vi "Host.vi"() -> ()   [LabVIEW 2018]
uses:
  <vilib>/userdefined/High Color/nirio_resource_hc.ctl
  <instrlib>/niDCPower/nidcpower.llb/niDCPower Measurement Type.ctl
  <vilib>/FPGAPlugInAG/PXI-7953R/niLvFpga_Open_PXI-7953R.vi
  <vilib>/rvi/interface/common/dynamic/niFpgaDynamicAddResources.vi
  <vilib>/FPGAPlugInAG/Dynamic/niLvFpga_Reset_Dynamic.vi
  <vilib>/FPGAPlugInAG/Dynamic/niLvFpga_Run_Dynamic.vi
  <vilib>/rvi/interface/common/niFpgaWaitOnOcc.vi
  <vilib>/Utility/error.llb/Error Cluster From Error Code.vi
  <vilib>/rvi/errors/niLvFpgaAdjustHostInterfaceError.vi
  <vilib>/FPGAPlugInAG/Dynamic/niLvFpga_Close_Dynamic.vi
  <vilib>/rvi/interface/nirviOpenFPGA/nirviOpenFPGA.xnode
  FPGA Bitfiles/7YLZHMM.lvbitx
  <vilib>/rvi/interface/nirviMethod/nirviMethod.xnode
  <vilib>/rvi/interface/nirviReadWriteControl/nirviReadWriteControl.xnode
  <vilib>/rvi/interface/nirviCloseFPGA/nirviCloseFPGA.xnode
  NiFpgaLv.dll
  <vilib>/rvi/interface/Simulation/niFpgaSimulationCallBeginRW.vi
  <vilib>/rvi/errors/niLvFpgaMergeErrorWithErrorCode.vi
  <vilib>/FPGAPlugInAG/Dynamic/niLvFpga_ConfigureFifo_Dynamic.vi
  <vilib>/FPGAPlugInAG/Dynamic/niLvFpga_WriteFifo_Dynamic.vi
panel:
  in  "SAVE":bool
  in  "FRAMES":path=path "C:/VPL/LabView_PRJ/Сериалайзер/FRAMES"
  in  "81920":u32=81920
  in  "Питание":bool
  in  "514":u16=514
  out "Записали FIFO":bool
  in  "Видео":bool
  in  "Запись!":bool
  in  "641":u16=641
  in  "512":u16=512
  in  "650":u16=650
  in  "File Path":path=path "C:/VPL/LabView_PRJ/Сериалайзер/EXAMPLES/Безымянныйййййййй.bmp"
  out "IFP":T1(plugin-control)
  in  "SER, V":dbl=3.3 caption="voltage level" format="%_6p"
  in  "SER_curlim":dbl=0.1 caption="current limit" format="%_6p"
  out "SER_cur":dbl caption="measurement" format="%_6g"
  out "ADC_char":dbl(graph)=5.2477070057568625e-05
  in  "1":refnum<k15>="PXI1Slot2"
  in  "FPGA":T2="PXI1Slot6"
  in  "СТОП":bool
  in  "Interface Name":string="NICFGen"
  out "Image":T1(plugin-control)
  out "Image Pixels (U32)":u32[][](array[numeric])
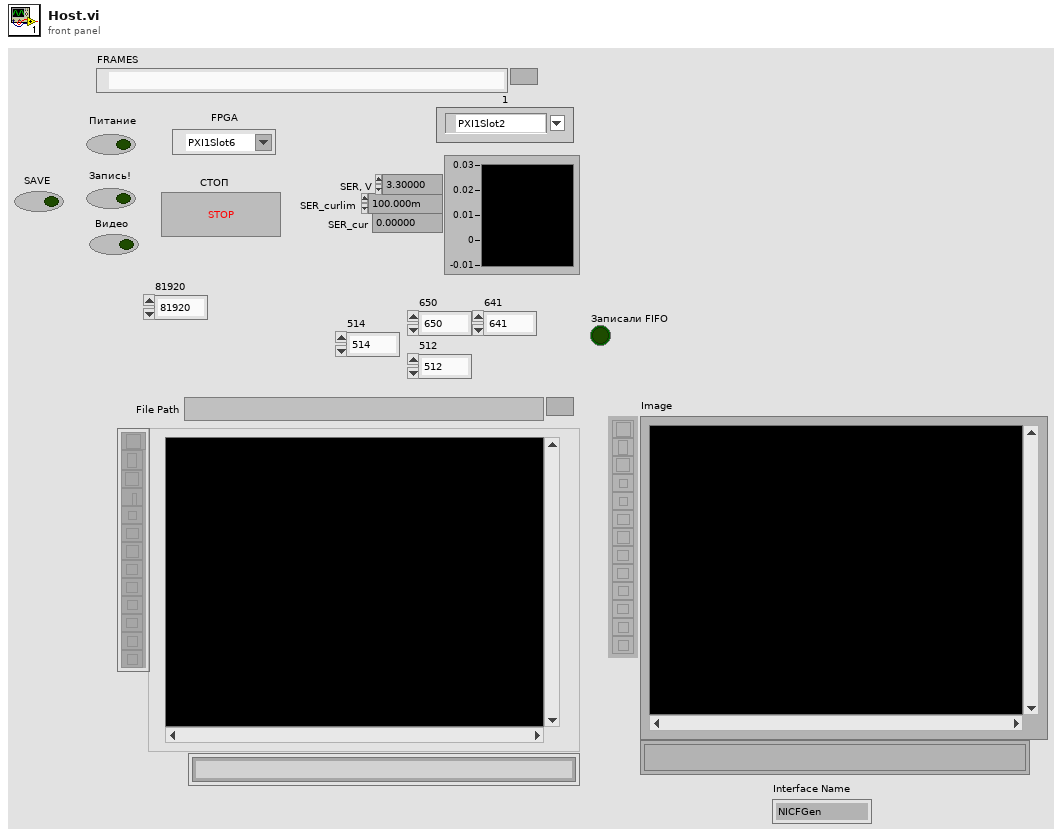
[diagram p1: front panel]
types:
  T1 = typedef "IMAQ Image.ctl" = refnum<image>
  T2 = typedef "nirio_resource_hc.ctl" = tag
  T3 = typedef "Image Type" = u32
  T4 = typedef "niDCPower Measurement Type.ctl" = i32
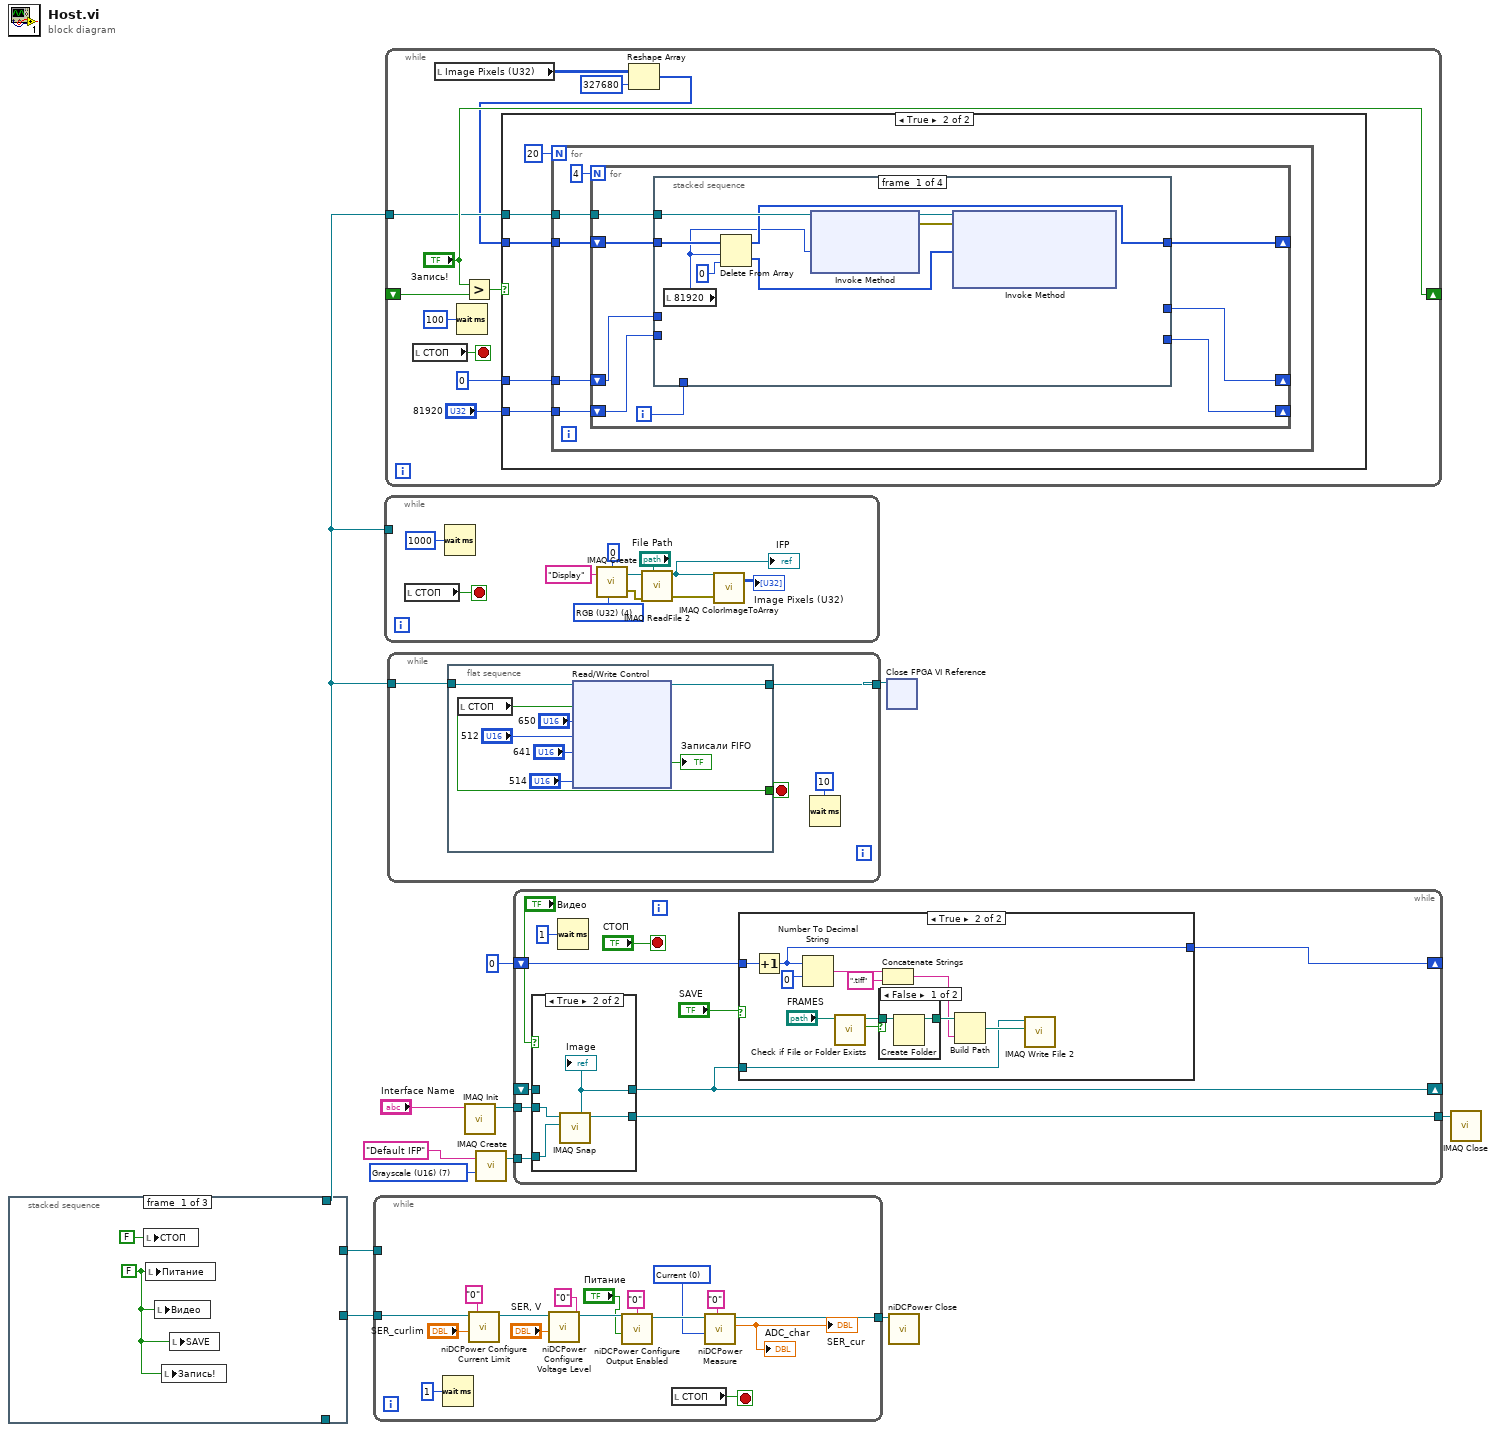
[diagram p0: block diagram]
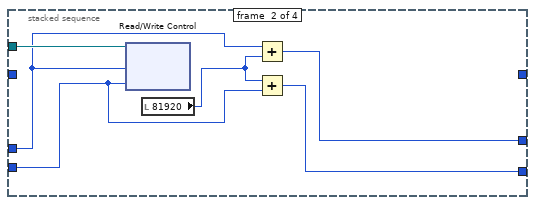
[diagram p6: hidden frame]
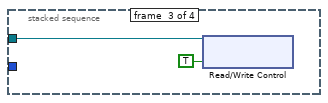
[diagram p7: hidden frame]
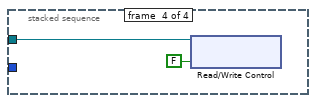
[diagram p8: hidden frame]
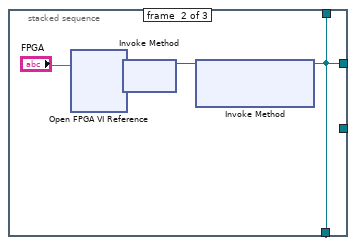
[diagram p9: hidden frame]
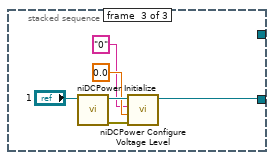
[diagram p10: hidden frame]
diagram:
  w5 = T3 7 items=["Grayscale (U8)", "Grayscale (I16)", "Grayscale (SGL)", "Complex (CSG)", "RGB (U32)", "HSL (U32)", "RGB (U64)", "Grayscale (U16)"] ("Image Type")
  n1 = stacked-sequence {
    tunnel: [_ w16 _] -> w10
    tunnel: [_ w16 _] -> w8
    tunnel: [_ w16 _] -> _
    tunnel: [_ _ w20] -> w12
    frame #0 {
      w13 = FALSE ("Питание")
      n2 = local write "СТОП"(FALSE ("СТОП")) -> ()
      n3 = local write "Питание"(w13) -> ()
      n4 = local write "Видео"(w13) -> ()
      n5 = local write "Запись!"(w13) -> ()
      n6 = local write "SAVE"(w13) -> ()
    }
    frame #1 {
      n7 = xnode "Open FPGA VI Reference"("resource name"="FPGA") -> ("FPGA VI Reference Out"=w18:refnum<k20>, "error out"=w17:errorcluster)  [unwired: 1 in]
      n8 = xnode "Invoke Method"("FPGA VI Reference In"=w18, "error in"=w17) -> ("FPGA VI Reference Out"=w15:refnum<k20>)  [unwired: 1 out]
      n9 = xnode "Invoke Method"("FPGA VI Reference In"=w15) -> ("FPGA VI Reference Out"=w16:refnum<k20>)  [unwired: 2 in, 1 out]
    }
    frame #2 {
      n10 = call <instrlib>:"niDCPower Initialize.vi"("resource name"="1") -> ("error out"=w25:errorcluster, "instrument handle out"=w24:refnum<k15>)  [unwired: 3 in, 6 out]
      n11 = call <instrlib>:"niDCPower Configure Voltage Level.vi"("error in (no error)"=w25, "voltage level"=0.0, "channel name"="0", "instrument handle"=w24) -> ("instrument handle out"=w20:refnum<k15>)  [unwired: 6 in, 1 out]
    }
  }
  n12 = while {
    tunnel: w12 -> [w28]
    tunnel: [w27] -> w11
    tunnel: w10 -> [_]
    stop <- w30 stop-if-true
    w34 = T4 0 items=["Current", "Voltage"] ("measurement type")
    n13 = Wait (ms)(milliseconds to wait=u32 1) -> ()  [unwired: 1 out]
    n14 = call <instrlib>:"niDCPower Configure Current Limit.vi"("current limit"="SER_curlim", "channel name"="0", "instrument handle"=w28) -> ("instrument handle out"=w38:refnum<k15>)  [unwired: 7 in, 1 out]
    n15 = call <instrlib>:"niDCPower Configure Voltage Level.vi"("voltage level"="SER, V", "channel name"="0", "instrument handle"=w38) -> ("instrument handle out"=w40:refnum<k15>)  [unwired: 7 in, 1 out]
    n16 = call <instrlib>:"niDCPower Configure Output Enabled.vi"("output enabled"="Питание", "channel name"="0", "instrument handle"=w40) -> ("instrument handle out"=w41:refnum<k15>)  [unwired: 7 in, 1 out]
    n17 = local read "СТОП"() -> (w30:bool)
    n18 = call <instrlib>:"niDCPower Measure.vi"("measurement type"=w34, "channel name"="0", "instrument handle"=w41) -> ("measurement"=→"SER_cur" →"ADC_char":dbl, "instrument handle out"=w27:refnum<k15>)  [unwired: 6 in, 1 out]
  }
  n19 = while {
    tunnel: w8 -> [_]
    stop <- w51 stop-if-true
    w44 = T3 4 items=["Grayscale (U8)", "Grayscale (I16)", "Grayscale (SGL)", "Complex (CSG)", "RGB (U32)", "HSL (U32)", "RGB (U64)", "Grayscale (U16)"] ("Image Type")
    n20 = local read "СТОП"() -> (w51:bool)
    n21 = Wait (ms)(milliseconds to wait=u32 1000) -> ()  [unwired: 1 out]
    n22 = call "IMAQ Create"("Border Size"=0, "Image Name"="Display", "Image Type"=w44) -> ("New Image"=w48:T1, "error out"=w45:errorcluster)  [unwired: 2 in]
    n23 = call "IMAQ ReadFile 2"("File Path"="File Path", "error in (no error)"=w45, "Image"=w48) -> ("error out"=w46:errorcluster, "Image Out"=w43:T1)  [unwired: 4 in, 3 out]
    "IFP" <- w43
    n24 = call "IMAQ ColorImageToArray"("Image"=w43, "error in (no error)"=w46) -> ("Image Pixels (U32)"=→"Image Pixels (U32)":u32[][])  [unwired: 2 in, 2 out]
  }
  n25 = while {
    shift-right: ["Запись!"] -> _
    shift-left: _ -> [w62]
    tunnel: w8 -> [w59]
    stop <- w63 stop-if-true
    n26 = local read "СТОП"() -> (w63:bool)
    n27 = local read "Image Pixels (U32)"() -> (w54:u32[][])
    n28 = Wait (ms)(milliseconds to wait=u32 100) -> ()  [unwired: 1 out]
    n29 = Greater?(x="Запись!", y=w62) -> (0:w60:bool)
    n30 = Reshape Array(w54, 327680 ("dimension size")) -> (w53:u32[])
    n31 = case shown="True" w60 {
      tunnel: w59 -> [_ w65]
      tunnel: "81920" -> [_ w68]
      tunnel: u32 0 ("length") -> [_ w67]
      tunnel: w53 -> [_ w66]
      frame False {
      }
      frame True {
        n32 = for {
          N: 20 -> [_]
          tunnel: w68 -> [w72]
          tunnel: w67 -> [w71]
          tunnel: w66 -> [w70]
          tunnel: w65 -> [w69]
          n33 = for {
            N: 4 -> [_]
            shift-right: [w78] -> _
            shift-left: w72 -> [w81]
            shift-right: [w79] -> _
            shift-left: w71 -> [w80]
            shift-right: [w76] -> _
            shift-left: w70 -> [w77]
            tunnel: w69 -> [w75]
            i -> [w74]
            n34 = stacked-sequence {
              tunnel: w75 -> [w88 w95 w97 w98]
              tunnel: w81 -> [_ w90 _ _]
              tunnel: w80 -> [_ w94 _ _]
              tunnel: [_ w93 _ _] -> w79
              tunnel: [_ w92 _ _] -> w78
              tunnel: w77 -> [w89 _ _ _]
              tunnel: [w87 _ _ _] -> w76
              tunnel: w74 -> [_ _ _ _]
              frame #0 {
                n35 = local read "81920"() -> (w82:u32)
                n36 = Delete From Array(array=w89, length=w82, index=0 ("length")) -> (deleted portion=w83:u32[], array with subset deleted=w87:u32[])
                n37 = xnode "Invoke Method"("FPGA VI Reference In"=w88, "Requested Depth"=w82) -> ("FPGA VI Reference Out"=w85:refnum<k20>, "error out"=w84:errorcluster)  [unwired: 1 in, 1 out]
                n38 = xnode "Invoke Method"("FPGA VI Reference In"=w85, "error in"=w84, "Data"=w83) -> ()  [unwired: 1 in, 3 out]
              }
              frame #1 {
                n39 = xnode "Read/Write Control"("FPGA VI Reference In"=w95, "Нач_адр"=w94, "Кон_адр"=w90) -> ()  [unwired: 1 in, 2 out]
                n40 = local read "81920"() -> (w91:u32)
                n41 = Add(x=w94, y=w91) -> (x+y=w93:u32)
                n42 = Add(x=w91, y=w90) -> (x+y=w92:u32)
              }
              frame #2 {
                n43 = xnode "Read/Write Control"("FPGA VI Reference In"=w97, "Кадр в ПЛИС"=TRUE) -> ()  [unwired: 1 in, 2 out]
              }
              frame #3 {
                n44 = xnode "Read/Write Control"("FPGA VI Reference In"=w98, "Кадр в ПЛИС"=FALSE) -> ()  [unwired: 1 in, 2 out]
              }
            }
          }
        }
      }
    }
  }
  n45 = while {
    tunnel: w8 -> [w103]
    tunnel: [w100] -> w9
    stop <- w102 stop-if-true
    n46 = flat-sequence {
      tunnel: w103 -> [w111]
      tunnel: [w105] -> w102
      tunnel: [w104] -> w100
      frame #0 {
        n47 = local read "СТОП"() -> (w105:bool)
        n48 = xnode "Read/Write Control"("FPGA VI Reference In"=w111, "СТОП!"=w105, "650"="650", "512"="512", "641"="641", "514"="514") -> ("FPGA VI Reference Out"=w104:refnum<k20>, "Записали FIFO"=→"Записали FIFO":bool)  [unwired: 1 in, 1 out]
      }
    }
    n49 = Wait (ms)(milliseconds to wait=u32 10) -> ()  [unwired: 1 out]
  }
  n50 = call <vilib>:"IMAQ Init.vi"("Interface Name"="Interface Name") -> ("IMAQ Session Out"=w2:refnum<k11>)  [unwired: 9 in, 1 out]
  n51 = call "IMAQ Create"("Image Name"="Default IFP", "Image Type"=w5) -> ("New Image"=w3:T1)  [unwired: 3 in, 1 out]
  n52 = while {
    tunnel: w3 -> [w119]
    tunnel: [w121] -> w7
    tunnel: w2 -> [w117]
    shift-right: [w113] -> _
    shift-left: _ -> [w116]
    shift-right: [w112] -> _
    shift-left: u32 0 -> [w114]
    stop <- "СТОП" stop-if-true
    n53 = case shown="True" "Видео" {
      tunnel: [w140 w142] -> w121
      tunnel: w117 -> [w140 w144]
      tunnel: w119 -> [_ w143]
      tunnel: [w139 w141] -> w113
      tunnel: w116 -> [w139 _]
      frame False {
      }
      frame True {
        n54 = call <vilib>:"IMAQ Snap.vi"("Image In"=w143, "IMAQ Session In"=w144) -> ("Image Out"=w141:T1, "IMAQ Session Out"=w142:refnum<k11>)  [unwired: 7 in, 1 out]
        "Image" <- w141
      }
    }
    n55 = Wait (ms)(milliseconds to wait=u32 1) -> ()  [unwired: 1 out]
    n56 = case shown="True" "SAVE" {
      tunnel: w114 -> [w123 w133]
      tunnel: w113 -> [_ w127]
      tunnel: [w123 w131] -> w112
      frame False {
      }
      frame True {
        n57 = Increment(x=w133) -> (x+1=w131:u32)
        n58 = Number To Decimal String(number=w131, width (-)=i16 0) -> (decimal integer string=w125:string)
        n59 = call <vilib>:"Check if File or Folder Exists.vi"("path"="FRAMES") -> ("file or folder exists?"=w134:bool, "dup path"=w135:path)  [unwired: 8 in, 1 out]
        n60 = case shown="False" w134 {
          tunnel: w135 -> [w137 w138]
          tunnel: [w136 w138] -> w129
          frame False {
            n61 = Create Folder(path (use dialog)=w137) -> (created path=w136:path)  [unwired: 2 in, 2 out]
          }
          frame True {
          }
        }
        n62 = Concatenate Strings(w125, ".tiff" ("string")) -> (w124:string)
        n63 = Build Path(base path=w129, name or relative path=w124) -> (appended path=w128:path)
        n64 = call-poly "IMAQ Write File 2"("File Path"=w128, "Image"=w127) -> ()  [unwired: 8 in, 2 out]
      }
    }
  }
  n65 = xnode "Close FPGA VI Reference"("FPGA VI Reference In"=w9) -> ()  [unwired: 1 in, 1 out]
  n66 = call <instrlib>:"niDCPower Close.vi"("instrument handle"=w11) -> ()  [unwired: 10 in, 1 out]
  n67 = call <vilib>:"IMAQ Close.vi"("IMAQ Session In"=w7) -> ()  [unwired: 10 in, 1 out]
